vi "Main.vi"() -> ()   [LabVIEW 2020, in "plugin_flodx_pressure.lvlib"]
doc: "pH Probe Plugin"
uses:
  plugin_flodx_pressure.lvlib
  plugin/process loops/Instrument Manager/loop/Instrument Loop State.ctl
  plugin/process loops/Instrument Manager/connection_info/Connection Info.ctl
  plugin/process loops/Instrument Manager/Instrument State.ctl
  plugin/process loops/UI Manager/Data Display Loop Data.ctl
  plugin/process loops/UI Manager/UI Data.ctl
  plugin/process loops/UI Manager/dialogs/settings/settings.ctl
  <userlib>/RxnRover/PluginCore/src/process loops/Acquisition/Acquisition Config.ctl
  plugin/process loops/Instrument Manager/Instrument Config.ctl
  <userlib>/RxnRover/PluginCore/src/process loops/Logging/loop/Logging Config.ctl
  <userlib>/RxnRover/PluginCore/src/process loops/Logging/log formats/Supported Log File Formats.ctl
  <userlib>/RxnRover/PluginCore/src/process loops/Logging/logger/Logging Start Mode.ctl
  <userlib>/RxnRover/PluginCore/src/process loops/Logging/logger/Logging Stop Mode.ctl
  plugin/process loops/System Control/System Control Data.ctl
  plugin/process loops/UI Manager/UI Display State.ctl
  56943c0d-d29c-4187-abe8-fcc35b9a4d89.vi
  aa3e49f4-ec9d-4bab-88e0-6a79f4e22ab8.vi
  <vilib>/Utility/error.llb/Error Cluster From Error Code.vi
  <vilib>/JDP Science/JSONtext/Variant to JSON Text.vi
  <vilib>/ErrorRing/Error Ring.xnode
  <vilib>/JDP Science/JSONtext/LVClass Serializer/JSONtext LVClass Serializer.lvclass
  <userlib>/RxnRover/PluginCore/src/support/Message Queue/Message Queue.lvlib
  plugin/plugin.lvlib
  <userlib>/RxnRover/PluginCore/src/process loops/Message Queues/Message Queues.lvlib
  <userlib>/RxnRover/PluginCore/src/support/User Event - Stop/User Event - Stop.lvlib
  plugin/process loops/Instrument Manager/Instrument Manager.lvlib
  <userlib>/RxnRover/PluginCore/src/process loops/Logging/Logging.lvlib
  <userlib>/RxnRover/PluginCore/src/process loops/Acquisition/Acquisition.lvlib
  <userlib>/RxnRover/PluginCore/src/process loops/Remote Connection Manager/Remote Connection Manager.lvlib
panel:
  out "Gauge Pressure":string
  out "Temperature":sgl
  out "Absolute":sgl
  out "Address":u8
  in  "Restart":bool
  out "Ambient":sgl
  in  "Open Calibrate Btn":bool
  out "Logging?":bool
  in  "Time Interval (sec)":i32=1200
  out "Data Graph":cluster{timestamp[], dbl[]}[](graph)
  in  "Open Settings Btn":bool
  in  "Toggle Logging":bool
  out "VISA resource":refnum<visa-resource-name>
  # "FloDx-Pressure Cer"
  # "Configuration"
  # "Device"
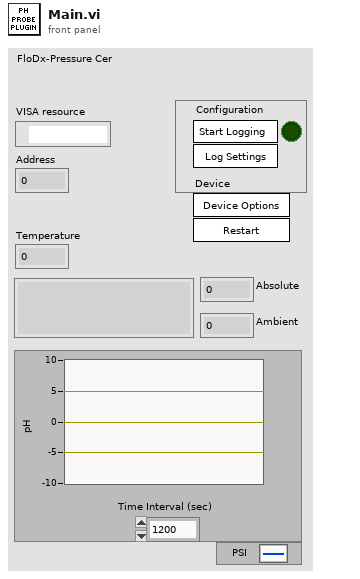
[diagram p1: front panel]
types:
  T1 = typedef "plugin_flodx_pressure.lvlib/plugin.lvlib/System Control Data.ctl" = cluster{"Example Value <Replace Me>":dbl, "Log Runs":bool, "Clone":bool}
  T2 = typedef "plugin_flodx_pressure.lvlib/plugin.lvlib/UI Data.ctl" = cluster{"UI Controls":cluster{"VISA Resource Ind":refnum<vi>, "Settings Btn":refnum<vi>, "Data Graph":refnum<vi>, "Logging Indicator":refnum<vi>, "Toggle Logging Btn":refnum<vi>, "Ambient Pressure":refnum<vi>, "Calibrate Btn":refnum<vi>, "Absolute Pressure":refnum<vi>, "Temperature":refnum<vi>, "Gauge Pressure":refnum<vi>}, "Plugin Settings":T3}
  T3 = typedef "plugin_flodx_pressure.lvlib/plugin.lvlib/settings.ctl" = cluster{"Acquisition Configuration":T4, "Instrument Configuration":T5, "Logging Configuration":T6, "Connection Info":T10}
  T4 = typedef "RxnRover_Plugin_Core.lvlib/Acquisition.lvlib/Acquisition Config.ctl" = cluster{"Query rate (sec)":dbl}
  T5 = typedef "plugin_flodx_pressure.lvlib/plugin.lvlib/Instrument Manager.lvlib/Instrument Config.ctl" = cluster{"Device":string, "Firmware Version":string}
  T6 = typedef "RxnRover_Plugin_Core.lvlib/Logging.lvlib/Logging Config.ctl" = cluster{"Log Directory":path, "Log File Format":T7, "Log File Name Prefix":string, "Logging Start Mode":T8, "Logging Stop Mode":T9, "Log Interval (Seconds)":dbl}
  T7 = typedef "RxnRover_Plugin_Core.lvlib/Logging.lvlib/Supported Log File Formats.ctl" = enum16{"Spreadsheet (CSV)"}
  T8 = typedef "RxnRover_Plugin_Core.lvlib/Logging.lvlib/Logging Start Mode.ctl" = enum16{"Manual Start", "Log While Running"}
  T9 = typedef "RxnRover_Plugin_Core.lvlib/Logging.lvlib/Logging Stop Mode.ctl" = enum16{"Log Continuously", "Log While Running"}
  T10 = typedef "plugin_flodx_pressure.lvlib/plugin.lvlib/Instrument Manager.lvlib/Connection Info.ctl" = cluster{"VISA Resource":refnum<visa-resource-name>, "Address":u8}
  T11 = typedef "plugin_flodx_pressure.lvlib/plugin.lvlib/Data Display Loop Data.ctl" = cluster{"Data Timestamps":timestamp[], "Data Values":dbl[], "Previous Run State":bool}
  T12 = typedef "plugin_flodx_pressure.lvlib/plugin.lvlib/Instrument Manager.lvlib/Instrument Loop State.ctl" = cluster{"Connection Info":T10, "Running":bool, "Running Since":timestamp, "Instrument State":T13}
  T13 = typedef "plugin_flodx_pressure.lvlib/plugin.lvlib/Instrument Manager.lvlib/Instrument State.ctl" = cluster{"Abs. Pressure":sgl, "Amb. Pressure":sgl, "Device":string, "Firmware Version":string, "Error Status":bool, "Error Code":i32, "Error Source":string, "Gauge Pressure":sgl, "Temperature":sgl, "Units (0-kPa,1-PSI,2-BAR)":dbl}
  T14 = typedef "RxnRover_Plugin_Core.lvlib/Message Queues.lvlib/All Message Queues.ctl" = cluster{"Acquisition":refnum<queue>, "Instrument":refnum<queue>, "Logging":refnum<queue>, "Remote":refnum<queue>, "System Control":refnum<queue>, "UI":refnum<queue>}
  T15 = typedef "plugin_flodx_pressure.lvlib/plugin.lvlib/UI Display State.ctl" = enum16{"Shown", "Hidden"}
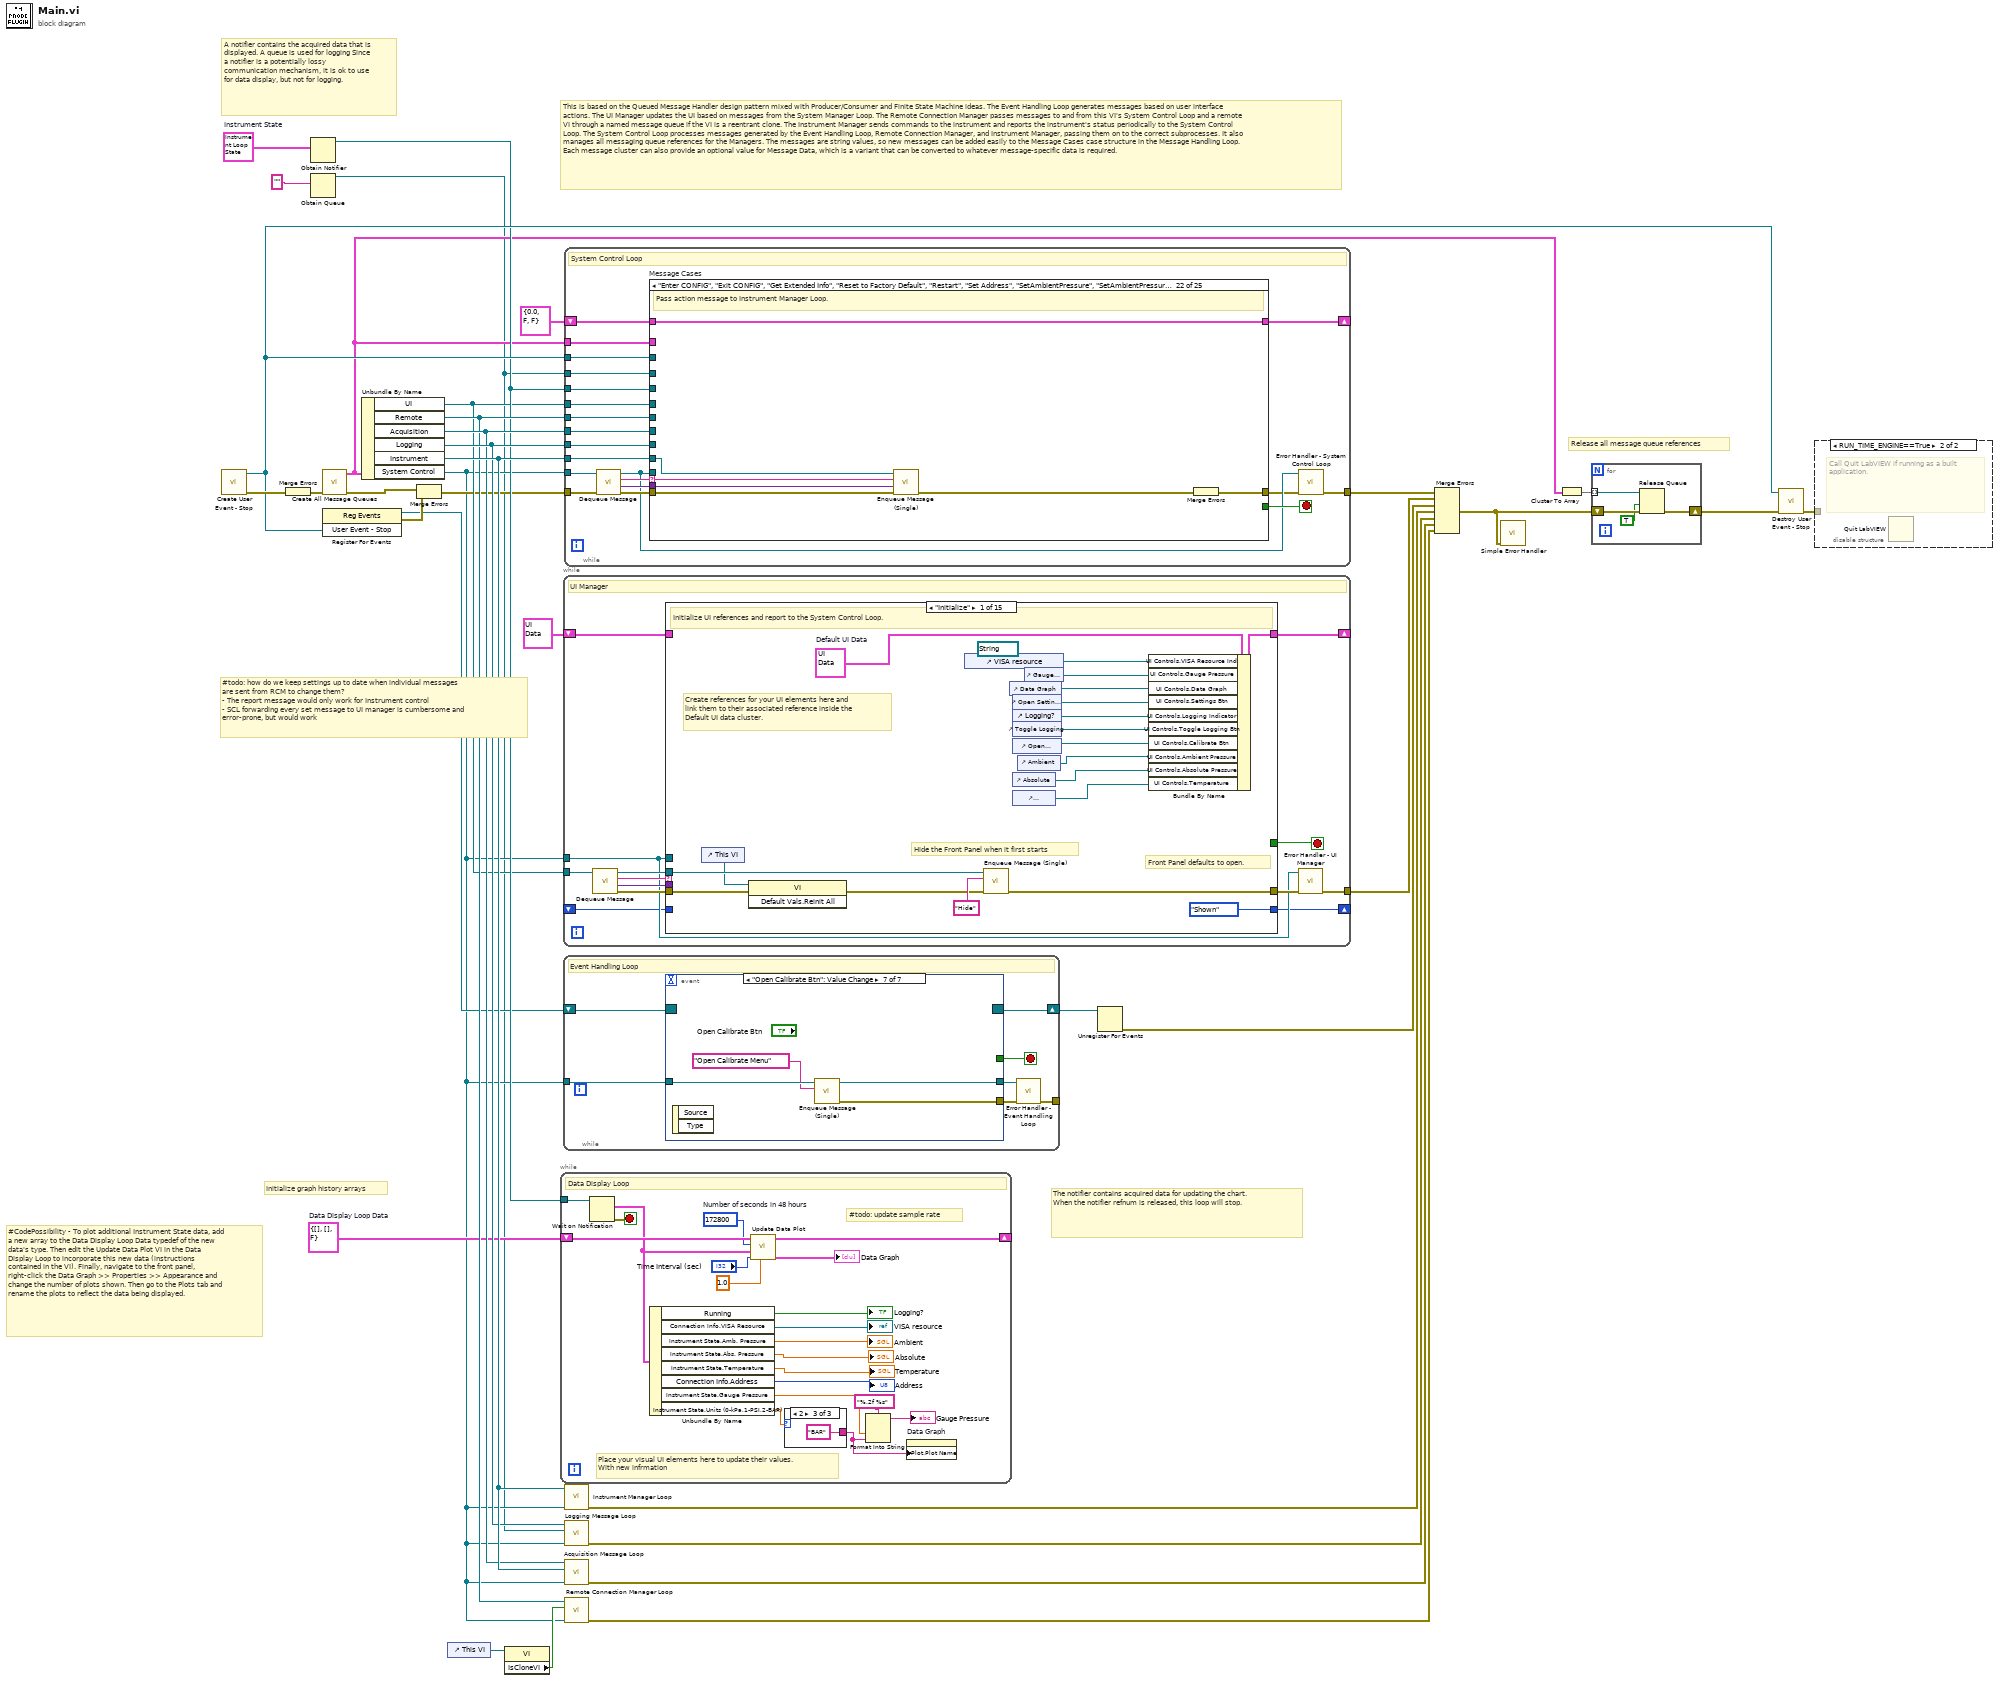
[diagram p0: block diagram]
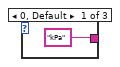
[diagram p2: hidden frame]
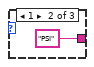
[diagram p3: hidden frame]
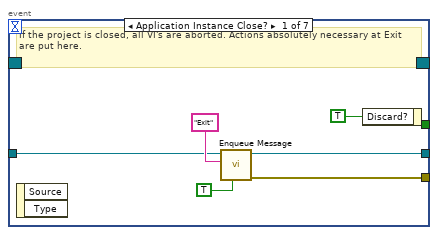
[diagram p4: hidden frame]
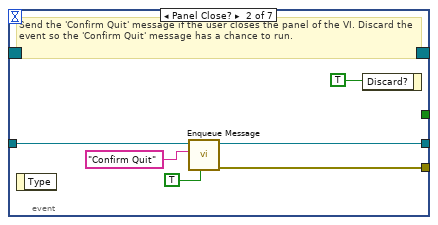
[diagram p5: hidden frame]
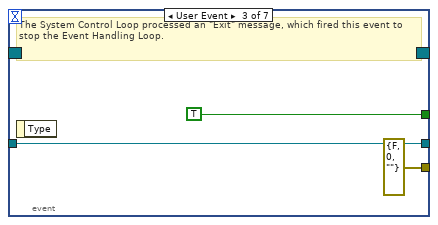
[diagram p6: hidden frame]
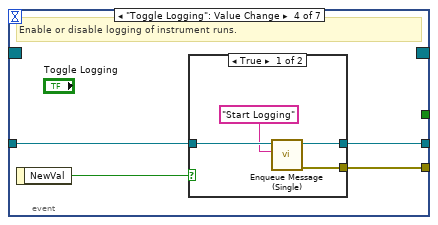
[diagram p7: hidden frame]
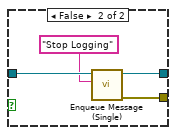
[diagram p8: hidden frame]
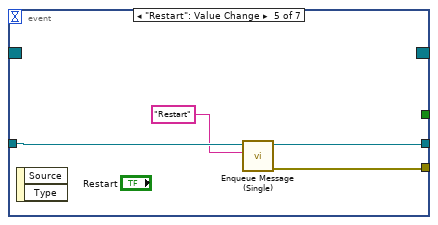
[diagram p9: hidden frame]
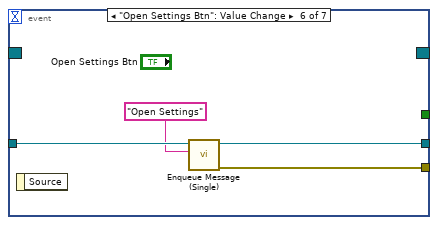
[diagram p10: hidden frame]
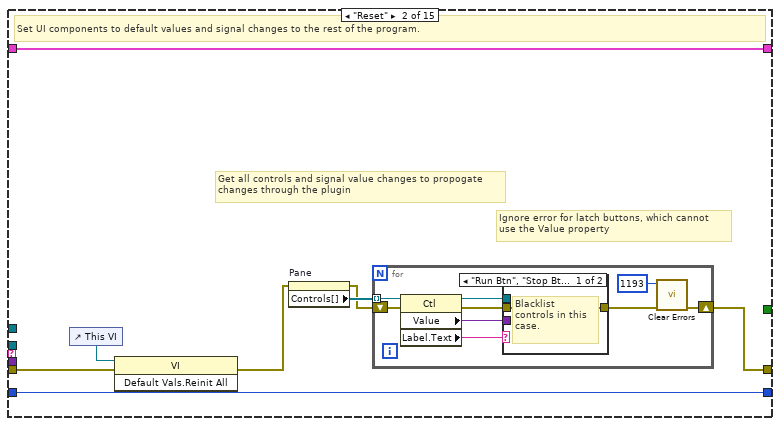
[diagram p11: hidden frame]
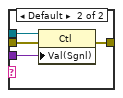
[diagram p12: hidden frame]
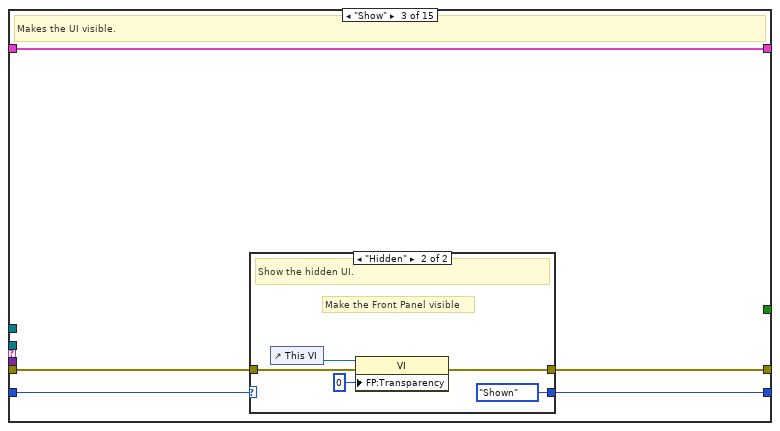
[diagram p13: hidden frame]
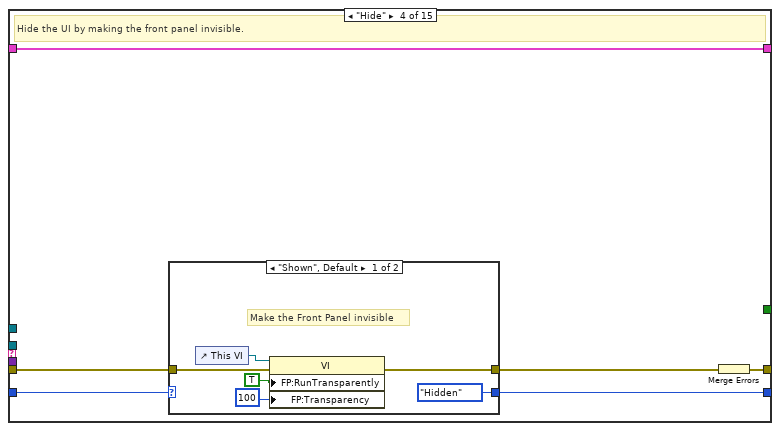
[diagram p15: hidden frame]
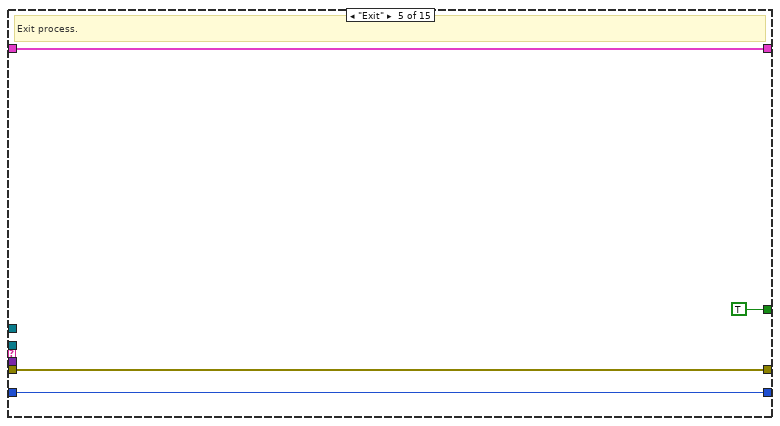
[diagram p17: hidden frame]
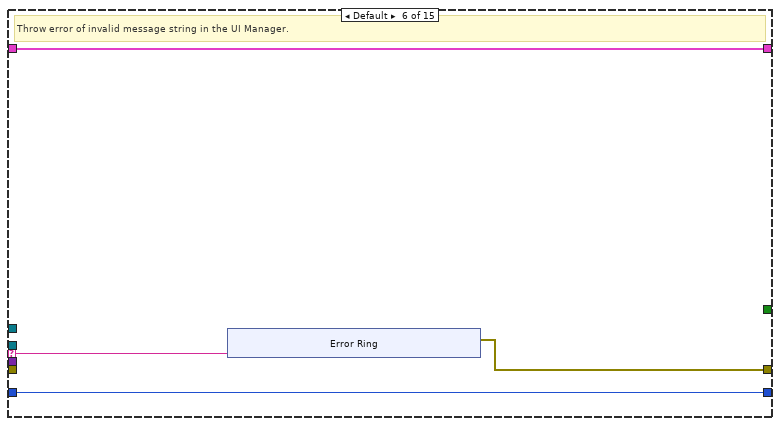
[diagram p18: hidden frame]
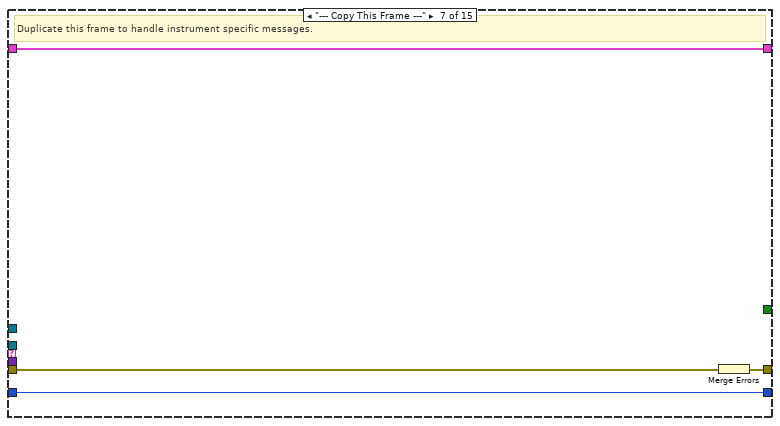
[diagram p19: hidden frame]
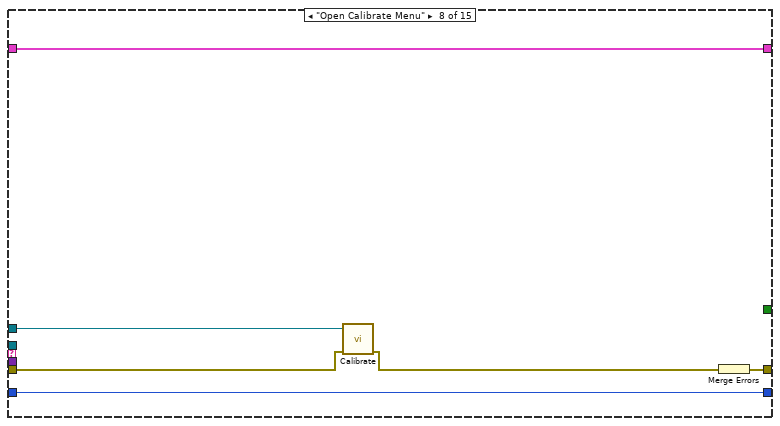
[diagram p20: hidden frame]
diagram:
  w9 = T11 {"Data Timestamps"=[], "Data Values"=[], "Previous Run State"=FALSE}  # Data Display Loop Data
  w12 = T12 {"Connection Info"={"VISA Resource"="", "Address"=1}, "Running"=FALSE, "Running Since"=timestamp(0 s since 1904-01-01), "Instrument State"={"Abs. Pressure"=0.0, "Amb. Pressure"=0.0, "Device"="", "Firmware Version"="", "Error Status"=FALSE, "Error Code"=0, "Error Source"="", "Gauge Pressure"=0.0, "Temperature"=0.0, "Units (0-kPa,1-PSI,2-BAR)"=0.0}}  # Instrument State
  # "#todo: how do we keep settings up to date when individual messages\nare sent from RCM to change them?\n- The report message would only work for Instrument control\n- SCL forwarding every set message to UI manager is cumbersome and\nerror-prone, but would work"
  # "#CodePossibility - To plot additional Instrument State data, add a new array to the Data Display Loop Data typedef of the new data's type. Then edit the Update Data Plot VI in the Data Display Loop to incorporate this new data (instructions contained in the VI). Finally, navigate to the front panel, right-click the Data Graph >> Properties >> Appearance and change the number of plots shown. Then go to the Plots tab and rename the plots to reflect the data being displayed."
  # "Initialize graph history arrays"
  # "A notifier contains the acquired data that is displayed. A queue is used for logging Since a notifier is a potentially lossy communication mechanism, it is ok to use for data display, but not for logging."
  # "The notifier contains acquired data for updating the chart. When the notifier refnum is released, this loop will stop."
  # "Release all message queue references"
  # "This is based on the Queued Message Handler design pattern mixed with Producer/Consumer and Finite State Machine ideas. The Event Handling Loop generates messages based on user interface actions. The UI Manager updates the UI based on messages from the System Manager Loop. The Remote Connection Manager passes messages to and from this VI's System Control Loop and a remote VI through a named message queue if the VI is a reentrant clone. The Instrument Manager sends commands to the instrument and reports the instrument's status periodically to the System Control Loop. The System Control Loop processes messages generated by the Event Handling Loop, Remote Connection Manager, and Instrument Manager, passing them on to the correct subprocesses. It also manages all messaging queue references for the Managers. The messages are string values, so new messages can be added easily to the Message Cases case structure in the Message Handling Loop.  Each message cluster can also provide an optional value for Message Data, which is a variant that can be converted to whatever message-specific data is required."
  n1 = call <userlib>:"Create User Event - Stop.vi"() -> ("error out"=w29:errorcluster, "User Event - Stop"=w25:refnum<user-event>)  [unwired: 10 in]
  n2 = Merge Errors(w29) -> (w28:errorcluster)
  n3 = Obtain Notifier(notification data type=w12) -> (notifier out=w13:refnum<notifier>)  [unwired: 3 in, 2 out]
  n4 = Obtain Queue(element data type="" ("<JSON>")) -> (queue out=w1:refnum<queue>)  [unwired: 4 in, 2 out]
  n5 = call <userlib>:"Create All Message Queues.vi"("error in (no error)"=w28) -> ("error out"=w31:errorcluster, "Message Queues out"=w7:T14)  [unwired: 9 in]
  n6 = register-events(w25) -> (reference out=w10:refnum<event-registration>, error out=w17:errorcluster)  [unwired: 2 in]
  n7 = Unbundle By Name(w7) -> ("UI"=w11:refnum<queue>, "Remote"=w32:refnum<queue>, "Acquisition"=w33:refnum<queue>, "Logging"=w34:refnum<queue>, "Instrument"=w35:refnum<queue>, "System Control"=w4:refnum<queue>)
  n8 = Merge Errors(w31, w17) -> (w5:errorcluster)
  n9 = control-ref of="This VI"() -> (w24:refnum<vi>)
  n10 = property class="VI"(reference=w24) -> ("IsCloneVI"=w23:bool)  [unwired: 1 in, 2 out]
  n11 = while "Data Display Loop" {
    tunnel: w13 -> [w55]
    shift-right: [w52] -> _
    shift-left: w9 -> [w53]
    stop <- w51 stop-if-true
    w48 = 172800  # Number of seconds in 48 hours
    # "Place your visual UI elements here to update their values.\nWith new infrmation"
    # "#todo: update sample rate"
    # "Data Display Loop"
    n12 = Wait on Notification(notifier=w55) -> (notification=w46:T12, error out=w51:errorcluster)  [unwired: 3 in, 2 out]
    n13 = Unbundle By Name(w46) -> ("Running"=→"Logging?":bool, "Connection Info.VISA Resource"=→"VISA resource":refnum<visa-resource-name>, "Instrument State.Amb. Pressure"=→"Ambient":sgl, "Instrument State.Abs. Pressure"=→"Absolute":sgl, "Instrument State.Temperature"=→"Temperature":sgl, "Connection Info.Address"=→"Address":u8, "Instrument State.Gauge Pressure"=w37:sgl, "Instrument State.Units (0-kPa,1-PSI,2-BAR)"=w41:dbl)
    n14 = call "Update Data Plot.vi"("Sample Rate (sec/sample)"=1.0, "Time interval (s)"="Time Interval (sec)", "Instrument State"=w46, "History length (-1; unlimited)"=w48, "Graph History Arrays in"=w53) -> ("Updated Plot History"=→"Data Graph":cluster{timestamp[], dbl[]}[], "Graph History Arrays out"=w52:T11)  [unwired: 5 in]
    n15 = case shown="2" w41 {
      tunnel: ["kPa" "PSI" "BAR"] -> w36
      frame 0, Default {
      }
      frame 1 {
      }
      frame 2 {
      }
    }
    n16 = Format Into String(format string="%.2f %s", w37, w36) -> (resulting string=→"Gauge Pressure":string)  [unwired: 2 in, 1 out]
    n17 = property on="Data Graph" class="XYGraph (strict)"("Plot.Plot Name"=w36) -> ()  [unwired: 2 in, 2 out]
  }
  n18 = while {
    tunnel: w11 -> [w71]
    tunnel: w4 -> [w62]
    tunnel: [w63] -> w22
    shift-right: [w66] -> _
    shift-left: T2 {"UI Controls"={"VISA Resource Ind"=refnum, "Settings Btn"=refnum, "Data Graph"=refnum, "Logging Indicator"=refnum, "Toggle Logging Btn"=refnum, "Ambient Pressure"=refnum, "Calibrate Btn"=refnum, "Absolute Pressure"=refnum, "Temperature"=refnum, "Gauge Pressure"=refnum}, "Plugin Settings"={"Acquisition Configuration"={"Query rate (sec)"=0.0}, "Instrument Configuration"={"Device"="", "Firmware Version"=""}, "Logging Configuration"={"Log Directory"=path "", "Log File Format"=enum."Spreadsheet (CSV)", "Log File Name Prefix"="", "Logging Start Mode"=enum."Manual Start", "Logging Stop Mode"=enum."Log Continuously", "Log Interval (Seconds)"=0.0}, "Connection Info"={"VISA Resource"="", "Address"=0}}} ("Default UI Data") -> [w65]
    shift-right: [w60] -> _
    shift-left: _ -> [w59]
    stop <- w61 stop-if-true
    # "UI Manager"
    n19 = call <userlib>:"Dequeue Message.vi"("Message Queue"=w71) -> ("error out"=w69:errorcluster, "Message Data"=w67:variant, "Message"=w68:string, "dup Message Queue"=w70:refnum<queue>)  [unwired: 7 in]
    n20 = case shown="\"Initialize\"" w68 {
      selector: w68 -> [_ _ _ _ _ w146 _ _ _ _ _ _ _ w220 _]
      tunnel: w70 -> [w87 _ _ _ _ _ _ _ _ _ _ _ _ _ _]
      tunnel: w69 -> [w81 w94 w116 w128 w142 _ w155 w159 w164 w167 w173 w182 w197 w219 w262]
      tunnel: w67 -> [_ _ _ _ _ _ _ _ _ _ _ _ _ w216 w252]
      tunnel: w62 -> [_ _ _ _ _ _ _ w160 _ _ _ _ w188 _ w257]
      tunnel: [w82 w93 w115 w129 w142 w145 w156 w162 w164 w167 w178 w187 w198 w215 w263] -> w64
      tunnel: [w89 w91 w117 w130 w141 w144 w157 w163 w165 w168 w176 w185 w194 w217 w259] -> w66
      tunnel: w65 -> [_ w91 w117 w130 w141 w144 w157 w163 w165 w168 w176 w185 w195 w214 w260]
      tunnel: [_ _ _ _ TRUE _ _ _ _ _ _ _ _ _ _] -> w61
      tunnel: w59 -> [_ w92 w114 w126 w139 w143 w154 w161 w166 w169 w177 w186 w196 w222 w261]
      tunnel: [UI_Display_State."Shown" ("UI Display State") w92 w113 w125 w139 w143 w154 w161 w166 w169 w177 w186 w196 w222 w261] -> w60
      frame "Initialize" {
        (unwired) refnum<vi> refnum ("Gauge Pressure")
        w90 = T2 {"UI Controls"={"VISA Resource Ind"=refnum, "Settings Btn"=refnum, "Data Graph"=refnum, "Logging Indicator"=refnum, "Toggle Logging Btn"=refnum, "Ambient Pressure"=refnum, "Calibrate Btn"=refnum, "Absolute Pressure"=refnum, "Temperature"=refnum, "Gauge Pressure"=refnum}, "Plugin Settings"={"Acquisition Configuration"={"Query rate (sec)"=0.0}, "Instrument Configuration"={"Device"="", "Firmware Version"=""}, "Logging Configuration"={"Log Directory"=path "", "Log File Format"=enum."Spreadsheet (CSV)", "Log File Name Prefix"="", "Logging Start Mode"=enum."Manual Start", "Logging Stop Mode"=enum."Log Continuously", "Log Interval (Seconds)"=0.0}, "Connection Info"={"VISA Resource"="", "Address"=0}}}  # Default UI Data
        # "Create references for your UI elements here and\nlink them to their associated reference inside the\nDefault UI data cluster."
        # "Front Panel defaults to open."
        # "Hide the Front Panel when it first starts"
        # "Initialize UI references and report to the System Control Loop."
        n21 = control-ref of="This VI"() -> (w83:refnum<vi>)
        n22 = invoke class="VI" method="Default Vals.Reinit All"(reference=w83, error in=w81) -> (error out=w80:errorcluster)  [unwired: 1 in, 2 out]
        n23 = control-ref of="VISA resource"() -> (w88:refnum<vi>)
        n24 = call <userlib>:"Enqueue Message (Single).vi"("error in (no error)"=w80, "Message"="Hide", "Message Queue"=w87) -> ("error out"=w82:errorcluster)  [unwired: 7 in, 1 out]
        n25 = control-ref of="Data Graph"() -> (w77:refnum<vi>)
        n26 = control-ref of="Open Settings Btn"() -> (w84:refnum<vi>)
        n27 = control-ref of="Logging?"() -> (w79:refnum<vi>)
        n28 = control-ref of="Toggle Logging"() -> (w78:refnum<vi>)
        n29 = control-ref of="Open Calibrate Btn"() -> (w76:refnum<vi>)
        n30 = control-ref of="Absolute"() -> (w74:refnum<vi>)
        n31 = control-ref of="Temperature"() -> (w73:refnum<vi>)
        n32 = control-ref of="Ambient"() -> (w75:refnum<vi>)
        n33 = control-ref of="Gauge Pressure"() -> (w72:refnum<vi>)
        n34 = Bundle By Name(cluster=w90, "UI Controls.VISA Resource Ind"=w88, "UI Controls.Gauge Pressure"=w72, "UI Controls.Data Graph"=w77, "UI Controls.Settings Btn"=w84, "UI Controls.Logging Indicator"=w79, "UI Controls.Toggle Logging Btn"=w78, "UI Controls.Calibrate Btn"=w76, "UI Controls.Ambient Pressure"=w75, "UI Controls.Absolute Pressure"=w74, "UI Controls.Temperature"=w73) -> (w89:T2)
      }
      frame "Reset" {
        # "Ignore error for latch buttons, which cannot\nuse the Value property"
        # "Get all controls and signal value changes to propogate\nchanges through the plugin"
        # "Set UI components to default values and signal changes to the rest of the program."
        n35 = control-ref of="This VI"() -> (w98:refnum<vi>)
        n36 = invoke class="VI" method="Default Vals.Reinit All"(reference=w98, error in=w94) -> (error out=w95:errorcluster)  [unwired: 1 in, 2 out]
        n37 = property on="Pane" class="Pane"(error in=w95) -> (error out=w96:errorcluster, "Controls[]"=w97:refnum<vi>[])  [unwired: 1 in, 1 out]
        n38 = for {
          tunnel: w97 -> [w107] mode=indexing
          shift-right: [w101] -> w93
          shift-left: w96 -> [w106]
          n39 = property class="Ctl"(reference=w107, error in=w106) -> (reference out=w105:refnum<vi>, error out=w104:errorcluster, "Value"=w103:variant, "Label.Text"=w99:string)
          n40 = case shown="\"Run Btn\", \"Stop Btn\"" w99 {
            tunnel: w105 -> [_ w112]
            tunnel: w104 -> [w108 w111]
            tunnel: w103 -> [_ w110]
            tunnel: [w108 w109] -> w102
            frame "Run Btn", "Stop Btn" {
              # "Blacklist controls in this case."
            }
            frame Default {
              n41 = property class="Ctl"(reference=w112, error in=w111, "Val(Sgnl)"=w110) -> (error out=w109:errorcluster)  [unwired: 1 out]
            }
          }
          n42 = call <vilib>:"Clear Errors.vi"("error in (no error)"=w102, "specific error code to clear (0: all)"=1193) -> ("error out"=w101:errorcluster)  [unwired: 4 in, 1 out]
        }
      }
      frame "Show" {
        # "Makes the UI visible."
        n43 = case shown="\"Hidden\"" w114 {
          selector: w114 -> [w119 _]
          tunnel: w116 -> [w118 w124]
          tunnel: [w118 w122] -> w115
          tunnel: [w119 UI_Display_State."Shown" ("UI Display State")] -> w113
          frame "Shown", Default {
            # "Do nothing if UI is already shown."
          }
          frame "Hidden" {
            # "Make the Front Panel visible"
            # "Show the hidden UI."
            n44 = control-ref of="This VI"() -> (w123:refnum<vi>)
            n45 = property class="VI"(reference=w123, error in=w124, "FP:Transparency"=u8 0 ("Front Panel Window:Transparency")) -> (error out=w122:errorcluster)  [unwired: 1 out]
          }
        }
      }
      frame "Hide" {
        # "Hide the UI by making the front panel invisible."
        n46 = case shown="\"Shown\", Default" w126 {
          selector: w126 -> [_ w138]
          tunnel: w128 -> [w133 w137]
          tunnel: [w132 w137] -> w127
          tunnel: [UI_Display_State."Hidden" ("UI Display State") w138] -> w125
          frame "Shown", Default {
            # "Make the Front Panel invisible"
            n47 = control-ref of="This VI"() -> (w136:refnum<vi>)
            n48 = property class="VI"(reference=w136, error in=w133, "FP:RunTransparently"=TRUE ("Front Panel Window:Run VI Transparently"), "FP:Transparency"=u8 100 ("Front Panel Window:Transparency")) -> (error out=w132:errorcluster)  [unwired: 1 out]
          }
          frame "Hidden" {
          }
        }
        n49 = Merge Errors(w127) -> (w129:errorcluster)
      }
      frame "Exit" {
        # "Exit process."
      }
      frame Default {
        # "Throw error of invalid message string in the UI Manager."
        n50 = xnode "Error Ring"("parameter 0"=w146) -> ("error out"=w145:errorcluster)
      }
      frame "--- Copy This Frame ---" {
        # "Duplicate this frame to handle instrument specific messages."
        n51 = Merge Errors(w155) -> (w156:errorcluster)
      }
      frame "Open Calibrate Menu" {
        n52 = call "Calibrate.vi"("error in (no error)"=w159, "Message Queue"=w160) -> ("error out"=w158:errorcluster)  [unwired: 9 in]
        n53 = Merge Errors(w158) -> (w162:errorcluster)
      }
      frame "Instrument Started" {
        # "The instrument started. Ensure that the UI reflects this."
      }
      frame "Instrument Stopped" {
        # "The instrument stopped. Ensure that the UI reflects this."
      }
      frame "Logging Started" {
        w170 = TRUE  # Logging is on
        # "Indicate that logging started."
        n54 = Unbundle By Name(w176) -> ("UI Controls.Logging Indicator"=w175:refnum<vi>, "UI Controls.Toggle Logging Btn"=w174:refnum<vi>)
        n55 = property class="Bool (strict)"(reference=w175, error in=w173, "Value"=w170) -> (error out=w172:errorcluster)  [unwired: 1 out]
        n56 = property class="Bool"(reference=w174, error in=w173, "Value"=w170) -> (error out=w171:errorcluster)  [unwired: 1 out]
        n57 = Merge Errors(w172, w171) -> (w178:errorcluster)
      }
      frame "Logging Stopped" {
        w179 = FALSE  # Logging is off
        # "Indicate that logging stopped."
        n58 = Unbundle By Name(w185) -> ("UI Controls.Logging Indicator"=w184:refnum<vi>, "UI Controls.Toggle Logging Btn"=w183:refnum<vi>)
        n59 = property class="Bool (strict)"(reference=w184, error in=w182, "Value"=w179) -> (error out=w181:errorcluster)  [unwired: 1 out]
        n60 = property class="Bool"(reference=w183, error in=w182, "Value"=w179) -> (error out=w180:errorcluster)  [unwired: 1 out]
        n61 = Merge Errors(w181, w180) -> (w187:errorcluster)
      }
      frame "Open Settings" {
        # "Open the settings dialog and send new settings to other loops"
        n62 = Unbundle By Name(w195) -> ("Plugin Settings"=w193:T3)
        n63 = call "Settings Dialog.vi"("error in (no error)"=w197, "System Control Queue"=w188, "Plugin Settings"=w193) -> ("error out"=w192:errorcluster, "Cancelled?"=w190:bool, "Plugin Settings out"=w189:T3)  [unwired: 6 in]
        n64 = case shown="False" w190 {
          tunnel: w192 -> [w204 w212]
          tunnel: [w211 w212] -> w191
          tunnel: w189 -> [w206 _]
          tunnel: w188 -> [w205 _]
          frame False {
            # "Settings dialog was not cancelled, send new settings"
            n65 = Unbundle By Name(w206) -> ("Acquisition Configuration"=w209:T4)
            n66 = Unbundle By Name(w206) -> ("Instrument Configuration"=w207:T5)
            n67 = Unbundle By Name(w206) -> ("Logging Configuration"=w202:T6)
            n68 = call <userlib>:"Enqueue Message (Single).vi"("error in (no error)"=w204, "Message Data"=w209, "Message"="New Acquisition Config", "Message Queue"=w205) -> ("error out"=w199:errorcluster)  [unwired: 6 in, 1 out]
            n69 = call <userlib>:"Enqueue Message (Single).vi"("error in (no error)"=w204, "Message Data"=w207, "Message"="New Instrument Config", "Message Queue"=w205) -> ("error out"=w200:errorcluster)  [unwired: 6 in, 1 out]
            n70 = call <userlib>:"Enqueue Message (Single).vi"("error in (no error)"=w204, "Message Data"=w202, "Message"="New Logging Config", "Message Queue"=w205) -> ("error out"=w201:errorcluster)  [unwired: 6 in, 1 out]
            n71 = Merge Errors(w199, w200, w201) -> (w211:errorcluster)
          }
          frame True {
            # "The settings dialog was cancelled, don't send anything"
          }
        }
        n72 = Bundle By Name(cluster=w195, "Plugin Settings"=w189) -> (w194:T2)
        n73 = Merge Errors(w191) -> (w198:errorcluster)
      }
      frame "Acquisition Config", "Instrument Config", "Logging Config" {
        # "Store the settings provided by another loop to display to the user"
        n74 = Scan From String(format string="%s Config", input string=w220, error in=w219) -> (error out=w213:errorcluster, output 1=w218:string)  [unwired: 2 in, 2 out]
        n75 = case shown="\"Acquisition\"" w218 {
          tunnel: w214 -> [w224 w231 w238 w245]
          tunnel: [w224 w230 w237 w244] -> w217
          tunnel: w216 -> [_ w229 w236 w242]
          tunnel: w213 -> [w223 w228 w235 w241]
          tunnel: [w223 w227 w232 w240] -> w215
          frame Default {
            # "I don't know how we would get here, but do nothing\nif an invalid string is given."
          }
          frame "Acquisition" {
            n76 = Variant To Data(error in=w228, type=T4 {"Query rate (sec)"=1.0} ("Acquisition Configuration"), Variant=w229) -> (data=w226:T4, error out=w227:errorcluster)
            n77 = Bundle By Name(cluster=w231, "Plugin Settings.Acquisition Configuration"=w226) -> (w230:T2)
          }
          frame "Instrument" {
            n78 = Variant To Data(error in=w235, type=T5 {"Device"="", "Firmware Version"=""} ("Instrument Configuration"), Variant=w236) -> (data=w233:T5, error out=w232:errorcluster)
            n79 = Bundle By Name(cluster=w238, "Plugin Settings.Instrument Configuration"=w233) -> (w237:T2)
          }
          frame "Logging" {
            n80 = Variant To Data(error in=w241, type=T6 {"Log Directory"=path "", "Log File Format"=enum."Spreadsheet (CSV)", "Log File Name Prefix"="experiment_", "Logging Start Mode"=enum."Manual Start", "Logging Stop Mode"=enum."Log Continuously", "Log Interval (Seconds)"=0.001} ("Logging Configuration"), Variant=w242) -> (data=w239:T6, error out=w240:errorcluster)
            n81 = Bundle By Name(cluster=w245, "Plugin Settings.Logging Configuration"=w239) -> (w244:T2)
          }
        }
      }
      frame "Get Connection Info" {
        # "Open the dialog to get connection info and send the new connection info back to the instrument manager to try"
        n82 = Unbundle By Name(w260) -> ("Plugin Settings.Connection Info"=w256:T10, "UI Controls.VISA Resource Ind"=w249:refnum<vi>)
        n83 = Variant To Data(error in=w262, type=errorcluster {"status"=FALSE, "code"=0, "source"=""} ("error out"), Variant=w252) -> (data=w251:errorcluster, error out=w254:errorcluster)
        n84 = call "Get Connection Information Dialog.vi"("error in (no error)"=w254, "previous attempt error (no error)"=w251, "Connection Info"=w256) -> ("error out"=w247:errorcluster, "Cancelled?"=w255:bool, "Connection Info out"=w250:T10)  [unwired: 6 in]
        n85 = Unbundle By Name(w250) -> ("VISA Resource"=w248:refnum<visa-resource-name>)
        n86 = property class="VISAName"(reference=w249, error in=w247, "Value"=w248) -> (error out=w246:errorcluster)  [unwired: 1 out]
        n87 = case shown="False" w255 {
          tunnel: w247 -> [w265 w273]
          tunnel: [w268 w272] -> w258
          tunnel: w250 -> [w264 _]
          tunnel: w257 -> [w266 w270]
          frame False {
            # "if not cancelled, send new connection info"
            n88 = call <userlib>:"Enqueue Message (Single).vi"("error in (no error)"=w265, "Message Data"=w264, "Message"="Set Connection Info", "Message Queue"=w266) -> ("error out"=w268:errorcluster)  [unwired: 6 in, 1 out]
          }
          frame True {
            # "If the user cancels the connection,\nclose the plugin."
            n89 = call <userlib>:"Enqueue Message (Single).vi"("Priority Message? (F)"=TRUE, "error in (no error)"=w273, "Message"="Exit", "Message Queue"=w270) -> ("error out"=w272:errorcluster)  [unwired: 6 in, 1 out]
          }
        }
        n90 = Bundle By Name(cluster=w260, "Plugin Settings.Connection Info"=w250) -> (w259:T2)
        n91 = Merge Errors(w246, w258) -> (w263:errorcluster)
      }
    }
    n92 = call "Error Handler - UI Manager.vi"("error in (no error)"=w64, "Message Queue"=w62) -> ("dup error in"=w63:errorcluster)  [unwired: 8 in, 1 out]
  }
  n93 = while {
    tunnel: w4 -> [w280]
    shift-right: [w278] -> w26
    shift-left: w10 -> [w279]
    tunnel: [w274] -> _
    stop <- w276 stop-if-true
    # "Event Handling Loop"
    n94 = event shown="[6] \"Open Calibrate Btn\": Value Change" {
      selector: w279 -> [_ _ _ _ _ _ _]
      dyn-events: [_ _ _ _ _ _ _] -> w278
      timeout: _ -> [_ _ _ _ _ _ _]
      tunnel: [_ _ TRUE ("Discard?") _ _ _ _] -> w276
      tunnel: w280 -> [w283 w291 w295 w299 w311 w315 w317]
      tunnel: [w281 w290 errorcluster {"status"=FALSE, "code"=0, "source"=""} ("error out") w296 w309 w312 w319] -> w277
      tunnel: [w282 w289 w295 w298 w310 w314 w318] -> w275
      event Application Instance Close? {
        # "If the project is closed, all VI's are aborted. Actions absolutely necessary at Exit are put here."
        n95 = event-data() -> ()  [unwired: 1 in, 2 out]
        n96 = call-poly <userlib>:"Enqueue Message.vi"("Priority Message? (F)"=TRUE, "Message"="Exit", "Message Queue"=w283) -> ("error out"=w281:errorcluster, "dup Message Queue"=w282:refnum<queue>)  [unwired: 7 in]
        n97 = event-data("Discard?"=TRUE) -> ()  [unwired: 1 in, 1 out]
      }
      event Panel Close? {
        # "Send the 'Confirm Quit' message if the user closes the panel of the VI. Discard the event so the 'Confirm Quit' message has a chance to run."
        n98 = event-data() -> ()  [unwired: 1 in, 1 out]
        n99 = call-poly <userlib>:"Enqueue Message.vi"("Priority Message? (F)"=TRUE, "Message"="Confirm Quit", "Message Queue"=w291) -> ("error out"=w290:errorcluster, "dup Message Queue"=w289:refnum<queue>)  [unwired: 7 in]
        n100 = event-data("Discard?"=TRUE) -> ()  [unwired: 1 in, 1 out]
      }
      event User Event {
        # "The System Control Loop processed an \"Exit\" message, which fired this event to stop the Event Handling Loop."
        n101 = event-data() -> ()  [unwired: 1 in, 1 out]
      }
      event "Toggle Logging": Value Change {
        # "Enable or disable logging of instrument runs."
        n102 = event-data() -> ("NewVal"=w297:bool)  [unwired: 1 in]
        n103 = case shown="True" w297 {
          tunnel: w299 -> [w303 w307]
          tunnel: [w302 w306] -> w298
          tunnel: [w300 w304] -> w296
          frame True {
            n104 = call <userlib>:"Enqueue Message (Single).vi"("Message"="Start Logging", "Message Queue"=w303) -> ("error out"=w300:errorcluster, "dup Message Queue"=w302:refnum<queue>)  [unwired: 8 in]
          }
          frame False {
            n105 = call <userlib>:"Enqueue Message (Single).vi"("Message"="Stop Logging", "Message Queue"=w307) -> ("error out"=w304:errorcluster, "dup Message Queue"=w306:refnum<queue>)  [unwired: 8 in]
          }
        }
      }
      event "Restart": Value Change {
        n106 = event-data() -> ()  [unwired: 1 in, 2 out]
        n107 = call <userlib>:"Enqueue Message (Single).vi"("Message"="Restart", "Message Queue"=w311) -> ("error out"=w309:errorcluster, "dup Message Queue"=w310:refnum<queue>)  [unwired: 8 in]
      }
      event "Open Settings Btn": Value Change {
        n108 = event-data() -> ()  [unwired: 1 in, 1 out]
        n109 = call <userlib>:"Enqueue Message (Single).vi"("Message"="Open Settings", "Message Queue"=w315) -> ("error out"=w312:errorcluster, "dup Message Queue"=w314:refnum<queue>)  [unwired: 8 in]
      }
      event "Open Calibrate Btn": Value Change {
        n110 = event-data() -> ()  [unwired: 1 in, 2 out]
        n111 = call <userlib>:"Enqueue Message (Single).vi"("Message"="Open Calibrate Menu", "Message Queue"=w317) -> ("error out"=w319:errorcluster, "dup Message Queue"=w318:refnum<queue>)  [unwired: 8 in]
      }
    }
    n112 = call "Error Handler - Event Handling Loop.vi"("error in (no error)"=w277, "Message Queue"=w275) -> ("dup error in"=w274:errorcluster)  [unwired: 8 in, 1 out]
  }
  n113 = while {
    tunnel: w4 -> [w331]
    shift-right: [w338] -> _
    shift-left: T1 {"Example Value <Replace Me>"=0.0, "Log Runs"=FALSE, "Clone"=FALSE} ("Default Data") -> [w339]
    tunnel: w25 -> [w336]
    tunnel: w5 -> [w335]
    tunnel: [w329] -> w30
    tunnel: w35 -> [w327]
    tunnel: w32 -> [w326]
    tunnel: w11 -> [w325]
    tunnel: w33 -> [w324]
    tunnel: w34 -> [w323]
    tunnel: w13 -> [w322]
    tunnel: w1 -> [w321]
    tunnel: w7 -> [w320]
    stop <- w337 stop-if-true
    # "System Control Loop"
    n114 = call <userlib>:"Dequeue Message.vi"("error in (no error)"=w335, "Message Queue"=w331) -> ("error out"=w334:errorcluster, "Message Data"=w332:variant, "Message"=w333:string, "dup Message Queue"=w330:refnum<queue>)  [unwired: 6 in]
    n115 = case "Message Cases" shown="\"Enter CONFIG\", \"Exit CONFIG\", \"Get Extended Info\", \"Reset to Factory Default\", \"Restart\", \"Set Address\", \"SetAmbientPressure\", \"SetAmbientPressureToCurrent\", \"SetUnits\", \"Start Instrument\", \"Stop Instrument\"" w333 {
      selector: w333 -> [_ _ _ w381 w394 w405 w423 _ w473 w480 w487 _ w526 w536 w543 w550 w563 w568 w576 w585 w599 w610 w621 w646 _]
      tunnel: w330 -> [w340 _ w361 _ _ _ _ w436 _ _ _ _ _ _ _ _ _ _ _ _ _ _ _ _ _]
      tunnel: w334 -> [w343 w358 w365 _ _ w408 w426 w441 w476 w483 w495 w523 w528 w539 w546 w553 w565 w572 w579 w588 w603 w613 _ w640 w648]
      tunnel: [w342 w352 w363 w384 w395 w414 w428 w438 w477 w484 w501 w522 w533 w540 w547 w554 w566 w573 w580 w589 w601 w614 w620 w638 w648] -> w328
      tunnel: w339 -> [_ w357 w364 w380 w396 w415 w429 w449 w475 w482 w500 w524 w534 w541 w548 w555 w567 w574 w581 w590 w602 w615 w619 w644 w649]
      tunnel: [w344 w357 w364 w380 w396 w415 w429 w449 w475 w482 w500 w524 w534 w541 w548 w555 w567 w574 w581 w590 w602 w615 w619 w644 w649] -> w338
      tunnel: [_ _ _ TRUE _ _ _ _ _ _ _ _ _ _ _ _ _ _ _ _ _ _ _ _ _] -> w337
      tunnel: w332 -> [_ w356 _ w385 _ w404 w422 w440 w472 w479 w488 w519 _ w537 w544 w551 w561 w569 w577 w586 w598 w611 w622 w634 _]
      tunnel: w336 -> [_ _ _ w382 _ _ _ _ _ _ _ _ _ _ _ _ _ _ _ _ _ _ _ _ _]
      tunnel: w327 -> [_ _ _ w377 _ w409 _ _ _ w478 _ _ _ _ _ _ _ _ _ _ _ w609 _ _ _]
      tunnel: w326 -> [_ _ _ w376 _ w412 w427 _ _ _ w505 _ _ _ _ _ _ _ _ w584 _ _ w623 _ _]
      tunnel: w325 -> [_ _ _ w375 _ w411 _ _ w471 _ w504 w521 _ w535 w542 w549 _ _ _ w583 _ _ w616 _ _]
      tunnel: w324 -> [_ _ _ w379 _ w413 _ _ _ _ w506 _ _ _ _ _ _ _ w575 _ w597 _ w618 _ _]
      tunnel: w323 -> [_ _ _ w378 _ w410 _ _ _ _ w497 _ w531 _ _ _ _ w570 _ _ _ _ w617 _ _]
      tunnel: w322 -> [_ _ _ w372 _ _ _ _ _ _ _ _ _ _ _ _ _ _ _ _ _ _ _ w643 _]
      tunnel: w321 -> [_ _ _ w370 _ _ _ _ _ _ _ _ _ _ _ _ _ _ _ _ _ _ _ w641 _]
      tunnel: w320 -> [_ _ _ _ _ _ _ _ _ _ _ _ _ _ _ _ w556 _ _ _ _ _ _ w635 _]
      frame "Initialize" {
        w345 = T1 {"Example Value <Replace Me>"=0.0, "Log Runs"=FALSE, "Clone"=FALSE}  # Default Data
        # "Initialize the system control loop and system."
        n116 = control-ref of="This VI"() -> ()  [unwired: 1 out]
        n117 = property on="Property Node" class="VI"() -> ("IsCloneVI"=w341:bool)  [unwired: 2 in, 2 out]
        n118 = Bundle By Name(cluster=w345, "Clone"=w341) -> (w344:T1)
        n119 = case shown="False" w341 {
          tunnel: w343 -> [w349 w351]
          tunnel: [w348 w351] -> w342
          tunnel: w340 -> [w347 _]
          frame False {
            # "Ask the user for connection info if this isn't a reentrant clone"
            n120 = call <userlib>:"Enqueue Message (Single).vi"("error in (no error)"=w349, "Message Data"=errorcluster {"status"=FALSE, "code"=0, "source"=""} ("error out"), "Message"="Get Connection Info", "Message Queue"=w347) -> ("error out"=w348:errorcluster)  [unwired: 6 in, 1 out]
          }
          frame True {
            # "Reentrant clone. It is the responsibility of the RCM to send the connection info command."
          }
        }
      }
      frame "Error" {
        # "#CodeRecommended - If you ever change the name of this \"Error\" message, you'll need to update the name in the Check Loop Error.vi as well."
        # "#CodeRecommended - Consider creating a system for logging errors in some way. These errors are for notification purposes only. Handling of specific errors should be performed in the message frames that generated the error."
        # "Error - Display an error dialog. This message is sent by the \"Error Handler\" VIs at the end of other loops in this application."
        n121 = Variant To Data(error in=w358, type=errorcluster {"status"=FALSE, "code"=0, "source"=""} ("error constant"), Variant=w356) -> (data=w354:errorcluster, error out=w353:errorcluster)
        n122 = call <vilib>:"Simple Error Handler.vi"("error in (no error)"=w354) -> ()  [unwired: 4 in, 5 out]
        n123 = Merge Errors(w353) -> (w352:errorcluster)
      }
      frame "Confirm Quit" {
        # "#CodeNeeded - If you want to provide an \"Are you sure\" dialog (or some other notification) before the application exits, place that code here. This message is typically sent from a Panel Close? event."
        # "Confirm Quit - Message that can confirm whether or not the user wants to exit the application."
        n124 = call-poly <userlib>:"Enqueue Message.vi"("Priority Message? (F)"=TRUE, "error in (no error)"=w365, "Message"="Exit", "Message Queue"=w361) -> ("error out"=w362:errorcluster)  [unwired: 6 in, 1 out]
        n125 = Merge Errors(w362) -> (w363:errorcluster)
      }
      frame "Exit" {
        # "Order other processes to exit"
        # "Begin the application closing procedure by sending \"Exit\" commands to all running processes."
        n126 = Variant To Data(type=errorcluster {"status"=FALSE, "code"=0, "source"=""} ("error constant"), Variant=w385) -> (data=w386:errorcluster)  [unwired: 1 in, 1 out]
        n127 = Build Array(w375, w376, w379, w378, w377) -> (w374:refnum<queue>[])
        n128 = call <vilib>:"Clear Errors.vi"("error in (no error)"=w386, "specific error code to clear (0: all)"=5000) -> ("error out"=w367:errorcluster)  [unwired: 4 in, 1 out]
        n129 = call <vilib>:"Simple Error Handler.vi"("error in (no error)"=w367) -> ()  [unwired: 4 in, 5 out]
        n130 = for {
          tunnel: w381 -> [w392]
          tunnel: w374 -> [w391] mode=indexing
          shift-right: [w390] -> w383
          shift-left: _ -> [w389]
          n131 = call <userlib>:"Enqueue Message (Single).vi"("Priority Message? (F)"=TRUE, "Message"=w392, "Message Queue"=w391) -> ("error out"=w393:errorcluster)  [unwired: 7 in, 1 out]
          n132 = Merge Errors(w393, w389) -> (w390:errorcluster)
        }
        n133 = Release Notifier(notifier=w372) -> (error out=w371:errorcluster)  [unwired: 2 in, 2 out]
        n134 = Release Queue(queue=w370) -> (error out=w368:errorcluster)  [unwired: 2 in, 2 out]
        n135 = call <userlib>:"Fire User Event - Stop.vi"("User Event - Stop"=w382) -> ("error out"=w369:errorcluster)  [unwired: 10 in]
        n136 = Merge Errors(w369, w368, w371, w383) -> (w384:errorcluster)
      }
      frame Default {
        # "'Default' case only runs if there is a message that isn't defined in any of the other cases.  Output a programming error."
        n137 = xnode "Error Ring"("parameter 0"=w394) -> ("error out"=w395:errorcluster)
      }
      frame "---Copy This Frame---" {
        # "Sends the message to each process in the array."
        # "#CodeRecommended - Change connections to build an array of the processes that will receive this message"
        # "Duplicate this frame when creating new messages.  Change this comment in the duplicated frame to describe this message."
        n138 = Build Array(w411, w412, w413, w410, w409) -> (w406:refnum<queue>[])
        n139 = for {
          tunnel: w406 -> [w419] mode=indexing
          tunnel: w405 -> [w421]
          tunnel: w404 -> [w420]
          shift-right: [w418] -> w407
          shift-left: w408 -> [w416]
          n140 = call <userlib>:"Enqueue Message (Single).vi"("Message Data"=w420, "Message"=w421, "Message Queue"=w419) -> ("error out"=w417:errorcluster)  [unwired: 7 in, 1 out]
          n141 = Merge Errors(w417, w416) -> (w418:errorcluster)
        }
        n142 = Merge Errors(w407) -> (w414:errorcluster)
      }
      frame "Set Remote Queue" {
        # "Sends the message to each process in the array."
        # "Bounce this message back to the Remote Control Manager to set the remote queue to publish messages to."
        n143 = Build Array(w427) -> (w424:refnum<queue>[])
        n144 = for {
          tunnel: w424 -> [w433] mode=indexing
          tunnel: w423 -> [w435]
          tunnel: w422 -> [w434]
          shift-right: [w432] -> w425
          shift-left: w426 -> [w430]
          n145 = call <userlib>:"Enqueue Message (Single).vi"("Message Data"=w434, "Message"=w435, "Message Queue"=w433) -> ("error out"=w431:errorcluster)  [unwired: 7 in, 1 out]
          n146 = Merge Errors(w431, w430) -> (w432:errorcluster)
        }
        n147 = Merge Errors(w425) -> (w428:errorcluster)
      }
      frame "Set Visa Resource" {
        # "String is expected to be \"<visa_resource>\""
        # "Update the communication information of the instrument."
        n148 = Variant To Data(error in=w441, type="", Variant=w440) -> (data=w443:string, error out=w448:errorcluster)
        n149 = call "Deserialize Connection Info.vi"("error in (no error)"=w448, "Connection Info String"=w443) -> ("error out"=w442:errorcluster, "Deserialized Connection Info"=w447:T10)  [unwired: 8 in]
        n150 = call <vilib>:"Clear Errors.vi"("error in (no error)"=w442, "specific error code to clear (0: all)"=85) -> ("error out"=w445:errorcluster, "specific error cleared?"=w444:bool)  [unwired: 4 in]
        n151 = case shown="False" w444 {
          tunnel: w436 -> [w455 w469]
          tunnel: w447 -> [w454 _]
          tunnel: [w450 w467] -> w439
          tunnel: w445 -> [w453 w468]
          tunnel: w443 -> [w451 _]
          tunnel: w442 -> [_ w466]
          frame False {
            n152 = Empty String/Path?(string/path=w451) -> (empty?=w452:bool)
            n153 = case shown="True" w452 {
              tunnel: w455 -> [w459 w461]
              tunnel: w454 -> [w458 _]
              tunnel: [w456 w462] -> w450
              tunnel: w453 -> [w457 w463]
              frame False {
                n154 = call <userlib>:"Enqueue Message (Single).vi"("error in (no error)"=w457, "Message Data"=w458, "Message"="Set Connection Info", "Message Queue"=w459) -> ("error out"=w456:errorcluster)  [unwired: 6 in, 1 out]
              }
              frame True {
                # "Empty resource string means the user needs to provide the info."
                n155 = call <userlib>:"Enqueue Message (Single).vi"("error in (no error)"=w463, "Message Data"=errorcluster {"status"=FALSE, "code"=0, "source"=""} ("error out"), "Message"="Get Connection Info", "Message Queue"=w461) -> ("error out"=w462:errorcluster)  [unwired: 6 in, 1 out]
              }
            }
          }
          frame True {
            # "If error 85 occurred, then the connection info string was invalid because the Scan from String function failed. The error being returned should report the exact issue."
            n156 = call <userlib>:"Enqueue Message (Single).vi"("error in (no error)"=w468, "Message Data"=w466, "Message"="Invalid Connection Info", "Message Queue"=w469) -> ("error out"=w467:errorcluster)  [unwired: 6 in, 1 out]
          }
        }
        n157 = Merge Errors(w439) -> (w438:errorcluster)
      }
      frame "Get Connection Info" {
        # "Request connection information from the user."
        n158 = call <userlib>:"Enqueue Message (Single).vi"("error in (no error)"=w476, "Message Data"=w472, "Message"=w473, "Message Queue"=w471) -> ("error out"=w474:errorcluster)  [unwired: 6 in, 1 out]
        n159 = Merge Errors(w474) -> (w477:errorcluster)
      }
      frame "Set Connection Info" {
        # "Request connection information from the user."
        n160 = call <userlib>:"Enqueue Message (Single).vi"("error in (no error)"=w483, "Message Data"=w479, "Message"=w480, "Message Queue"=w478) -> ("error out"=w481:errorcluster)  [unwired: 6 in, 1 out]
        n161 = Merge Errors(w481) -> (w484:errorcluster)
      }
      frame "Valid Connection Info" {
        # "Convert before sending"
        # "When a Valid Communication Info has been chosen, start the other processes."
        n162 = Unbundle By Name(w500) -> ("Log Runs"=w499:bool)
        n163 = call "To JSON Text.vim"("error in (no error)"=w495, "Anything"=w488) -> ("error out"=w494:errorcluster, "<JSON>"=w493:string)  [unwired: 8 in]
        n164 = call <userlib>:"Enqueue Message (Single).vi"("error in (no error)"=w494, "Message Data"=w493, "Message"=w487, "Message Queue"=w497) -> ("error out"=w498:errorcluster, "dup Message Queue"=w496:refnum<queue>)  [unwired: 6 in]
        n165 = case shown="True" w499 {
          tunnel: w498 -> [w509 w513]
          tunnel: w496 -> [_ w512]
          tunnel: [w509 w510] -> w507
          frame False {
          }
          frame True {
            n166 = call <userlib>:"Enqueue Message (Single).vi"("error in (no error)"=w513, "Message"="Start", "Message Queue"=w512) -> ("error out"=w510:errorcluster)  [unwired: 7 in, 1 out]
          }
        }
        n167 = call <userlib>:"Enqueue Message (Single).vi"("error in (no error)"=w507, "Message"="Start", "Message Queue"=w506) -> ("error out"=w489:errorcluster)  [unwired: 7 in, 1 out]
        n168 = Unbundle By Name(w500) -> ("Clone"=w502:bool)
        n169 = Variant To Data(error in=w489, type=T10 {"VISA Resource"="", "Address"=1} ("Connection Info"), Variant=w488) -> (data=w490:T10, error out=w486:errorcluster)
        n170 = call "Serialize Connection Info.vi"("error in (no error)"=w486, "Connection Info"=w490) -> ("error out 2"=w491:errorcluster, "Serialized Connection Info"=w492:string)  [unwired: 8 in]
        n171 = call <userlib>:"Enqueue Message (Single).vi"("error in (no error)"=w491, "Message Data"=w492, "Message"=w487, "Message Queue"=w505) -> ("error out"=w503:errorcluster)  [unwired: 6 in, 1 out]
        n172 = case shown="True" w502 {
          tunnel: w503 -> [w517 w518]
          tunnel: [w516 w518] -> w501
          tunnel: w504 -> [w515 _]
          frame False {
            # "Show the Front Panel automatically on startup"
            n173 = call <userlib>:"Enqueue Message (Single).vi"("error in (no error)"=w517, "Message"="Show", "Message Queue"=w515) -> ("error out"=w516:errorcluster)  [unwired: 7 in, 1 out]
          }
          frame True {
            # "Reentrant clone. It is the responsibility of the RCM to send \"Show\" if the plugin UI is desired."
          }
        }
      }
      frame "Invalid Connection Info" {
        # "On invalid connection info, ask the user to try to fix it."
        n174 = call <userlib>:"Enqueue Message (Single).vi"("error in (no error)"=w523, "Message Data"=w519, "Message"="Get Connection Info", "Message Queue"=w521) -> ("error out"=w522:errorcluster)  [unwired: 6 in, 1 out]
      }
      frame "Start Logging", "Stop Logging" {
        # "Extract if this is the start or stop command"
        # "Forward the message to start or stop logging."
        n175 = Scan From String(format string="%s Logging", input string=w526, error in=w528) -> (error out=w527:errorcluster, output 1=w525:string)  [unwired: 2 in, 2 out]
        n176 = call <userlib>:"Enqueue Message (Single).vi"("Priority Message? (F)"=TRUE, "error in (no error)"=w527, "Message"=w525, "Message Queue"=w531) -> ("error out"=w532:errorcluster)  [unwired: 6 in, 1 out]
        n177 = Merge Errors(w532) -> (w533:errorcluster)
      }
      frame "Open Settings" {
        # "Message to open the settings dialog."
        n178 = call <userlib>:"Enqueue Message (Single).vi"("error in (no error)"=w539, "Message Data"=w537, "Message"=w536, "Message Queue"=w535) -> ("error out"=w538:errorcluster)  [unwired: 6 in, 1 out]
        n179 = Merge Errors(w538) -> (w540:errorcluster)
      }
      frame "Open Calibrate Menu" {
        # "Message to open the settings dialog."
        n180 = call <userlib>:"Enqueue Message (Single).vi"("error in (no error)"=w546, "Message Data"=w544, "Message"=w543, "Message Queue"=w542) -> ("error out"=w545:errorcluster)  [unwired: 6 in, 1 out]
        n181 = Merge Errors(w545) -> (w547:errorcluster)
      }
      frame "Acquisition Config", "Instrument Config", "Logging Config" {
        # "#todo: This may get sent to RCM later"
        # "A process loop reporting its public config values."
        n182 = call <userlib>:"Enqueue Message (Single).vi"("error in (no error)"=w553, "Message Data"=w551, "Message"=w550, "Message Queue"=w549) -> ("error out"=w552:errorcluster)  [unwired: 6 in, 1 out]
        n183 = Merge Errors(w552) -> (w554:errorcluster)
      }
      frame "New Acquisition Config", "New Instrument Config", "New Logging Config" {
        # "Send new settings to the corresponding process loop."
        n184 = Scan From String(format string="New %s Config", input string=w563, error in=w565) -> (error out=w558:errorcluster, output 1=w562:string)  [unwired: 2 in, 2 out]
        n185 = call <userlib>:"Get Queue by Name.vi"("error in (no error)"=w558, "Queue Name"=w562, "Message Queues in"=w556) -> ("error out"=w557:errorcluster, "Queue out"=w559:refnum<queue>)  [unwired: 7 in]
        n186 = call <userlib>:"Enqueue Message (Single).vi"("error in (no error)"=w557, "Message Data"=w561, "Message"=w563, "Message Queue"=w559) -> ("error out"=w560:errorcluster)  [unwired: 6 in, 1 out]
        n187 = Merge Errors(w560) -> (w566:errorcluster)
      }
      frame "Set Entry Names", "Set Log Directory", "Set Log File Delimiter", "Set Log File Prefix", "Set Log on Run" {
        # "Pass on message to set a logging config value to the Logging Loop."
        n188 = call <userlib>:"Enqueue Message (Single).vi"("error in (no error)"=w572, "Message Data"=w569, "Message"=w568, "Message Queue"=w570) -> ("error out"=w571:errorcluster)  [unwired: 6 in, 1 out]
        n189 = Merge Errors(w571) -> (w573:errorcluster)
      }
      frame "Set Acquisition Messages" {
        # "Pass on message to set the acquisition messages."
        n190 = call <userlib>:"Enqueue Message (Single).vi"("error in (no error)"=w579, "Message Data"=w577, "Message"=w576, "Message Queue"=w575) -> ("error out"=w578:errorcluster)  [unwired: 6 in, 1 out]
        n191 = Merge Errors(w578) -> (w580:errorcluster)
      }
      frame "Logging Started", "Logging Stopped" {
        # "Pass on Logging status message to RCM and UI."
        n192 = Build Array(w583, w584) -> (w582:refnum<queue>[])
        n193 = for {
          tunnel: w586 -> [w593]
          tunnel: w585 -> [w592]
          shift-right: [w594] -> w587
          shift-left: w588 -> [w595]
          tunnel: w582 -> [w591] mode=indexing
          n194 = call <userlib>:"Enqueue Message (Single).vi"("error in (no error)"=w595, "Message Data"=w593, "Message"=w592, "Message Queue"=w591) -> ("error out"=w594:errorcluster)  [unwired: 6 in, 1 out]
        }
        n195 = Merge Errors(w587) -> (w589:errorcluster)
      }
      frame "Change Refresh" {
        # "Change the sampling rate of the instrument. Default value is the default set on the front panel control."
        n196 = Build Array(w597) -> (w596:refnum<queue>[])
        n197 = for {
          tunnel: w599 -> [w606]
          tunnel: w598 -> [w605]
          tunnel: w596 -> [w604] mode=indexing
          shift-right: [w607] -> w600
          shift-left: w603 -> [w608]
          n198 = call <userlib>:"Enqueue Message (Single).vi"("error in (no error)"=w608, "Message Data"=w605, "Message"=w606, "Message Queue"=w604) -> ("error out"=w607:errorcluster)  [unwired: 6 in, 1 out]
        }
        n199 = Merge Errors(w600) -> (w601:errorcluster)
      }
      frame "Enter CONFIG", "Exit CONFIG", "Get Extended Info", "Reset to Factory Default", "Restart", "Set Address", "SetAmbientPressure", "SetAmbientPressureToCurrent", "SetUnits", "Start Instrument", "Stop Instrument" {
        # "Pass action message to Instrument Manager Loop."
        n200 = call <userlib>:"Enqueue Message (Single).vi"("error in (no error)"=w613, "Message Data"=w611, "Message"=w610, "Message Queue"=w609) -> ("error out"=w612:errorcluster)  [unwired: 6 in, 1 out]
        n201 = Merge Errors(w612) -> (w614:errorcluster)
      }
      frame "Instrument Started", "Instrument Stopped" {
        # "Build an array of all processes that will receive this message"
        # "Notify processes of update"
        # "Notify processes of the instrument run state change."
        n202 = Build Array(w616, w623, w618, w617) -> (w624:refnum<queue>[])
        n203 = for {
          tunnel: w624 -> [w628] mode=indexing
          tunnel: w621 -> [w630]
          tunnel: w622 -> [w629]
          shift-right: [w627] -> w620
          shift-left: _ -> [w625]
          n204 = call <userlib>:"Enqueue Message (Single).vi"("Message Data"=w629, "Message"=w630, "Message Queue"=w628) -> ("error out"=w626:errorcluster)  [unwired: 7 in, 1 out]
          n205 = Merge Errors(w626, w625) -> (w627:errorcluster)
        }
      }
      frame "Report" {
        # "Convert to RCM"
        # "Send instrument state notification"
        # "Notify processes that the instrument stopped running."
        n206 = Variant To Data(error in=w640, type=T12 {"Connection Info"={"VISA Resource"="", "Address"=1}, "Running"=FALSE, "Running Since"=timestamp(0 s since 1904-01-01), "Instrument State"={"Abs. Pressure"=0.0, "Amb. Pressure"=0.0, "Device"="", "Firmware Version"="", "Error Status"=FALSE, "Error Code"=0, "Error Source"="", "Gauge Pressure"=0.0, "Temperature"=0.0, "Units (0-kPa,1-PSI,2-BAR)"=0.0}} ("Instrument State"), Variant=w634) -> (data=w631:T12, error out=w639:errorcluster)
        n207 = Unbundle By Name(w635) -> ("Remote"=w647:refnum<queue>)
        n208 = call "To JSON Text.vim"("Anything"=w631) -> ("<JSON>"=w633:string)  [unwired: 9 in, 1 out]
        n209 = call "Convert to Remote Instrument State.vi"("Internal Instrument State in"=w631) -> ("Remote Instrument State out"=w632:variant)  [unwired: 9 in, 1 out]
        n210 = Enqueue Element(queue=w641, element=w633, error in (no error)=w639) -> (error out=w636:errorcluster)  [unwired: 1 in, 2 out]
        n211 = Send Notification(notification=w631, notifier=w643, error in (no error)=w639) -> (error out=w637:errorcluster)  [unwired: 1 out]
        n212 = call <userlib>:"Enqueue Message (Single).vi"("error in (no error)"=w639, "Message Data"=w632, "Message"=w646, "Message Queue"=w647) -> ("error out"=w645:errorcluster)  [unwired: 6 in, 1 out]
        n213 = Merge Errors(w636, w637, w645) -> (w638:errorcluster)
      }
      frame "Valid Port Mappings" {
        # "Notify processes that the instrument stopped running."
      }
    }
    n214 = call "Error Handler - System Control Loop.vi"("error in (no error)"=w328, "Message Queue"=w330) -> ("dup error in"=w329:errorcluster)  [unwired: 8 in, 1 out]
  }
  n215 = call "Instrument Manager Loop.vi"("System Control"=w4, "Instrument Manager"=w35) -> ("error out"=w20:errorcluster)  [unwired: 9 in]
  n216 = call <userlib>:"Logging Message Loop.vi"("System Control"=w4, "Data Queue"=w1, "Logging"=w34) -> ("error out"=w19:errorcluster)  [unwired: 8 in]
  n217 = call <userlib>:"Acquisition Message Loop.vi"("System Control"=w4, "Instrument Manager"=w35, "Acquisition"=w33) -> ("error out"=w18:errorcluster)  [unwired: 8 in]
  n218 = call <userlib>:"Remote Connection Manager Loop.vi"("System Control"=w4, "IsCloneVI (false)"=w23, "Remote"=w32) -> ("error out"=w8:errorcluster)  [unwired: 8 in]
  n219 = Unregister For Events(event registration refnum=w26) -> (error out=w21:errorcluster)  [unwired: 1 in]
  n220 = Merge Errors(w30, w22, w21, w20, w19, w18, w8) -> (w16:errorcluster)
  n221 = call <vilib>:"Simple Error Handler.vi"("error in (no error)"=w16) -> ()  [unwired: 4 in, 5 out]
  n222 = Cluster To Array(cluster=w7) -> (array=w15:refnum<queue>[])
  n223 = for {
    shift-right: [w651] -> w14
    shift-left: w16 -> [w652]
    tunnel: w15 -> [w653] mode=indexing
    n224 = Release Queue(queue=w653, force destroy? (F)=TRUE, error in (no error)=w652) -> (error out=w651:errorcluster)  [unwired: 2 out]
  }
  n225 = call <userlib>:"Destroy User Event - Stop.vi"("error in (no error)"=w14, "User Event - Stop"=w25) -> ("error out"=w27:errorcluster)  [unwired: 9 in]
  n226 = disable-structure shown="RUN_TIME_ENGINE==True" {
    disable-tunnel: w27 -> [_ _]
    frame condition #0 (active) {
    }
    frame condition #1 {
      # "Call Quit LabVIEW if running as a built application."
      n227 = Quit LabVIEW() -> ()  [unwired: 1 in]
    }
  }
